vi "Show Diagram.vi"(8 "error in (no error)":errorcluster, 11 "Module ID":i32=-1) -> (0 "error out":errorcluster)   [LabVIEW 2017, in "MQTT.lvlib"]
doc: "This VI tells the Module to show its block diagram to facilitate troubleshooting (add probes, breakpoints, highlight execution, etc).\n\n_____\nBased on Delacor QMH Project Template 3.1.0.34."
uses:
  MQTT.lvlib
  Show Diagram Argument--cluster.ctl
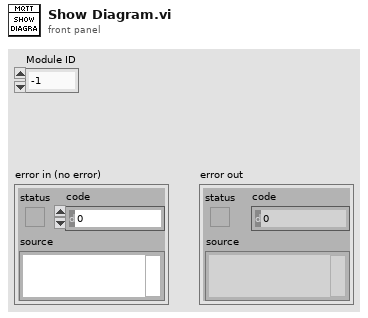
[diagram p1: front panel]
types:
  T1 = typedef "MQTT.lvlib/Show Diagram Argument--cluster.ctl" = cluster{"Module ID":i32, "Debug?":bool}
  T2 = typedef "MQTT.lvlib/Request Events--cluster.ctl" = cluster{"Stop Module":refnum<user-event>, "Show Panel":refnum<user-event>, "Hide Panel":refnum<user-event>, "Show Diagram":refnum<user-event>, "Get Module Execution Status":refnum<user-event>, "Configure":refnum<user-event>, "Connect":refnum<user-event>, "disconnect":refnum<user-event>, "Subscrie":refnum<user-event>, "unsubscribe":refnum<user-event>, "Publish":refnum<user-event>, "Register Event":refnum<user-event>, "broadcastTopic":refnum<user-event>}
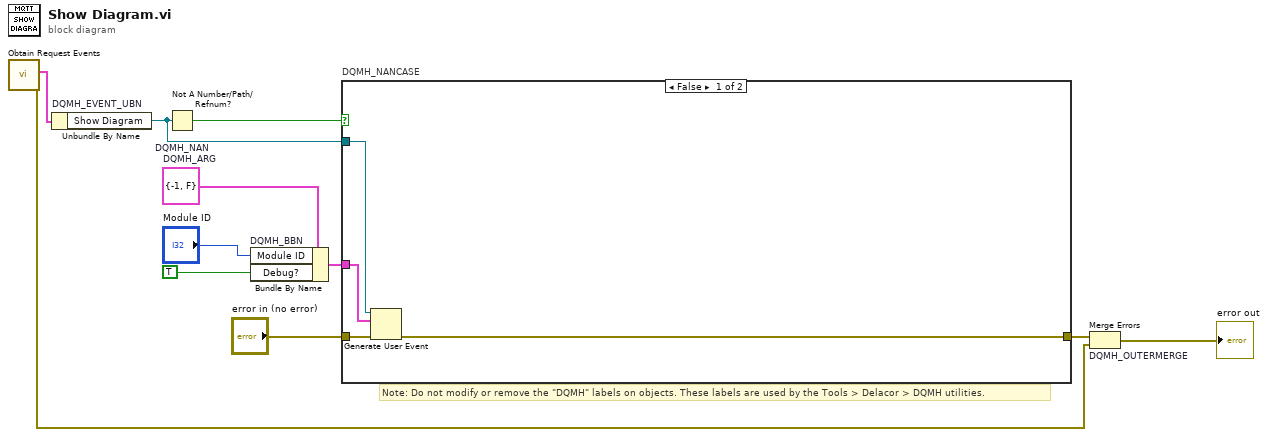
[diagram p0: block diagram]
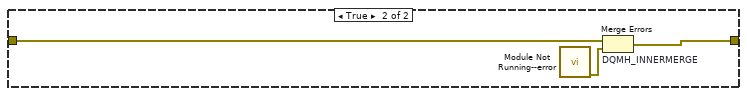
[diagram p2: hidden frame]
diagram:
  w5 = T1 {"Module ID"=-1, "Debug?"=FALSE}  # DQMH_ARG
  # "Note: Do not modify or remove the \"DQMH\" labels on objects. These labels are used by the Tools > Delacor > DQMH utilities."
  n1 = call "Obtain Request Events.vi"() -> ("error out"=w1:errorcluster, "MQTT Request Events"=w2:T2)  [unwired: 10 in]
  n2 = Unbundle By Name "DQMH_EVENT_UBN"(w2) -> ("Show Diagram"=w6:refnum<user-event>)
  n3 = Not A Number/Path/Refnum? "DQMH_NAN"(number/path/refnum=w6) -> (NaN/Path/Refnum?=w7:bool)
  n4 = Bundle By Name "DQMH_BBN"(cluster=w5, "Module ID"="Module ID", "Debug?"=TRUE) -> (w8:T1)
  n5 = case "DQMH_NANCASE" shown="False" w7 {
    tunnel: "error in (no error)" -> [w15 w18]
    tunnel: [w14 w17] -> w9
    tunnel: w6 -> [w13 _]
    tunnel: w8 -> [w12 _]
    frame False {
      n6 = Generate User Event(user event=w13, event data cluster=w12, error in=w15) -> (error out=w14:errorcluster)  [unwired: 1 in, 1 out]
    }
    frame True {
      n7 = call "Module Not Running--error.vi"() -> ("error out"=w16:errorcluster)  [unwired: 11 in]
      n8 = Merge Errors "DQMH_INNERMERGE"(w18, w16) -> (w17:errorcluster)
    }
  }
  n9 = Merge Errors "DQMH_OUTERMERGE"(w9, w1) -> (→"error out":errorcluster)
